vi "VFD FGV.vi"(4 "Slave ID (255)":u8, 5 "values Mutiple Reg":u16[](array[numeric]), 6 "State":T1, 7 "Coil Value":bool, 8 "error In":errorcluster, 9 "value":u16, 10 "address":u16, 11 "IP Address":string="localhost") -> (0 "error out":errorcluster, 2 "Coils":bool[](array[boolean]), 3 "Registers":u16[](array[numeric]))   [LabVIEW 2026, in "VFD Library.lvlib"]
uses:
  VFD Library.lvlib
  State Selection FGV.ctl
  <vilib>/NI/Modbus Library/API/Master/Modbus Master.lvclass
  <vilib>/NI/Modbus Library/API/Wrapper/Create TCP Master.vi
  <vilib>/NI/Modbus Library/API/Wrapper/API Main.lvlib
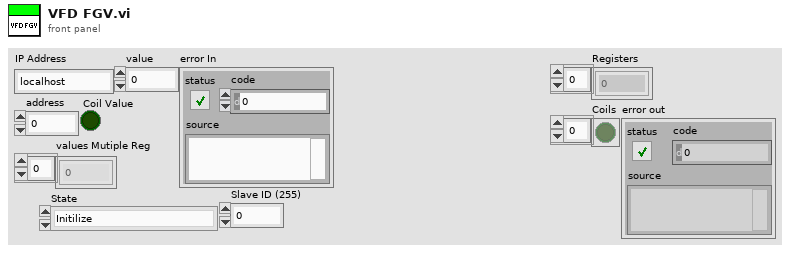
[diagram p1: front panel]
types:
  T1 = typedef "State Selection FGV.ctl" = enum16{"Initilize", "Write Reg", "Write Multiple Reg", "Read Reg", "Write Coil", "Read Coil", "Reset", "Close"}
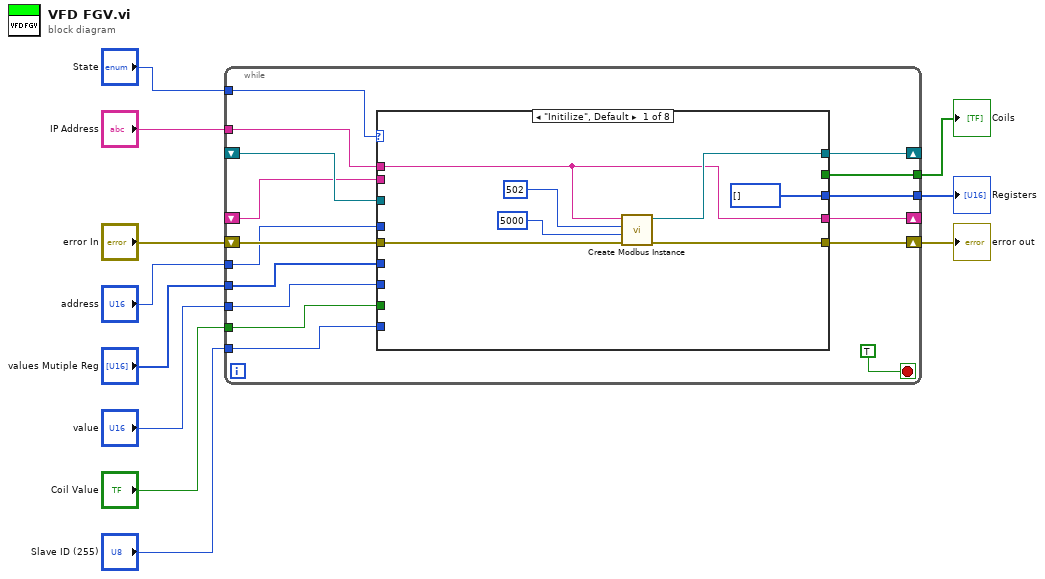
[diagram p0: block diagram]
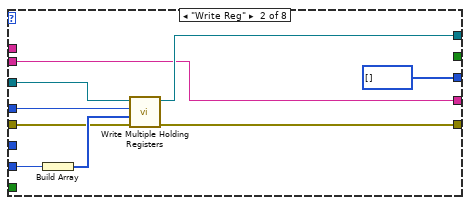
[diagram p2: hidden frame]
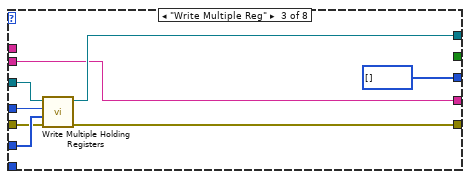
[diagram p3: hidden frame]
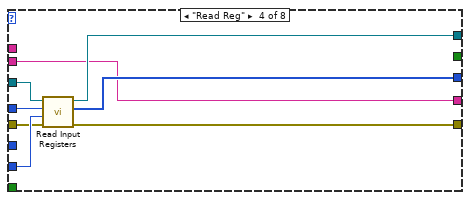
[diagram p4: hidden frame]
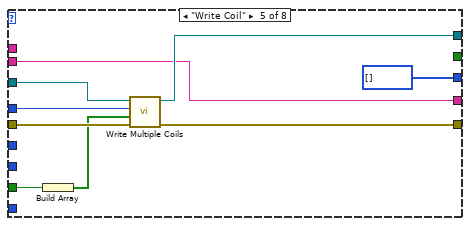
[diagram p5: hidden frame]
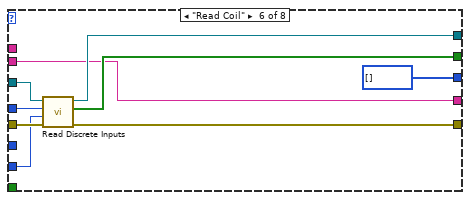
[diagram p6: hidden frame]
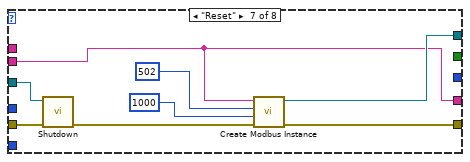
[diagram p7: hidden frame]
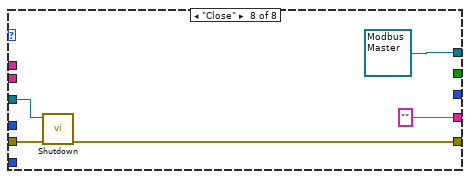
[diagram p8: hidden frame]
diagram:
  n1 = while {
    tunnel: "IP Address" -> [w26]
    shift-right: [w25] -> _
    shift-left: _ -> [w21]
    shift-right: [w24] -> w3
    shift-left: "error In" -> [w23]
    tunnel: "State" -> [w22]
    tunnel: "address" -> [w20]
    tunnel: "value" -> [w19]
    tunnel: [w18] -> w7
    tunnel: "Coil Value" -> [w17]
    tunnel: [w16] -> w5
    tunnel: "values Mutiple Reg" -> [w15]
    tunnel: "Slave ID (255)" -> [w14]
    shift-right: [w13] -> _
    shift-left: _ -> [w12]
    stop <- TRUE stop-if-true
    n2 = case shown="\"Initilize\", Default" w22 {
      tunnel: w26 -> [w28 _ _ _ _ _ _ _]
      tunnel: [w33 w38 w50 w58 w66 w75 w83 refnum<class "Modbus Master.lvclass"> refnum ("Modbus Master")] -> w25
      tunnel: [w31 w36 w45 w53 w64 w73 w82 w87] -> w24
      tunnel: w23 -> [w32 w37 w46 w55 w65 w74 w85 w88]
      tunnel: w21 -> [_ w39 w49 w59 w67 w76 w84 w89]
      tunnel: w20 -> [_ w42 w48 w57 w63 w71 _ _]
      tunnel: w19 -> [_ w41 _ w56 _ w70 _ _]
      tunnel: [u16[] [] ("Registers") u16[] [] ("Registers") u16[] [] ("Registers") w54 u16[] [] ("Registers") u16[] [] ("Registers") _ _] -> w18
      tunnel: w17 -> [_ _ _ _ w62 _ _ _]
      tunnel: [_ _ _ _ _ w72 _ _] -> w16
      tunnel: w15 -> [_ _ w47 _ _ _ _ _]
      tunnel: w14 -> [_ _ _ _ _ _ _ _]
      tunnel: [w28 w35 w44 w52 w60 w69 w79 "" ("IP Address")] -> w13
      tunnel: w12 -> [_ w35 w44 w52 w60 w69 w79 _]
      frame "Initilize", Default {
        n3 = call-poly <vilib>:"Create Modbus Instance.vi"("error in"=w32, "connect timeout ms"=5000 ("Timeout (10000)"), "port (502)"=u16 502 ("Port (502)"), "address"=w28) -> ("error out"=w31:errorcluster, "TCP master instance"=w33:refnum<class "Modbus Master.lvclass">)  [unwired: 6 in]
      }
      frame "Write Reg" {
        n4 = Build Array(w41) -> (w40:u16[])
        n5 = call-dynamic "Write Multiple Holding Registers.vi"("error in"=w37, "registers to write"=w40, "starting address"=w42, "Modbus master in"=w39) -> ("error out"=w36:errorcluster, "Modbus master out"=w38:refnum<class "Modbus Master.lvclass">)  [unwired: 6 in]
      }
      frame "Write Multiple Reg" {
        n6 = call-dynamic "Write Multiple Holding Registers.vi"("error in"=w46, "registers to write"=w47, "starting address"=w48, "Modbus master in"=w49) -> ("error out"=w45:errorcluster, "Modbus master out"=w50:refnum<class "Modbus Master.lvclass">)  [unwired: 6 in]
      }
      frame "Read Reg" {
        n7 = call-dynamic "Read Input Registers.vi"("error in"=w55, "number of inputs"=w56, "starting address"=w57, "Modbus master in"=w59) -> ("error out"=w53:errorcluster, "register values"=w54:u16[], "Modbus master out"=w58:refnum<class "Modbus Master.lvclass">)  [unwired: 5 in]
      }
      frame "Write Coil" {
        n8 = Build Array(w62) -> (w61:bool[])
        n9 = call-dynamic "Write Multiple Coils.vi"("error in"=w65, "coils to write"=w61, "starting address"=w63, "Modbus master in"=w67) -> ("error out"=w64:errorcluster, "Modbus master out"=w66:refnum<class "Modbus Master.lvclass">)  [unwired: 6 in]
      }
      frame "Read Coil" {
        n10 = call-dynamic "Read Discrete Inputs.vi"("error in"=w74, "number of inputs"=w70, "starting address"=w71, "Modbus master in"=w76) -> ("error out"=w73:errorcluster, "discrete inputs"=w72:bool[], "Modbus master out"=w75:refnum<class "Modbus Master.lvclass">)  [unwired: 5 in]
      }
      frame "Reset" {
        n11 = call-dynamic "Shutdown.vi"("error in"=w85, "Modbus master in"=w84) -> ("error out"=w81:errorcluster)  [unwired: 9 in]
        n12 = call-poly <vilib>:"Create Modbus Instance.vi"("error in"=w81, "connect timeout ms"=1000 ("Timeout (10000)"), "port (502)"=u16 502 ("Port (502)"), "address"=w79) -> ("error out"=w82:errorcluster, "TCP master instance"=w83:refnum<class "Modbus Master.lvclass">)  [unwired: 6 in]
      }
      frame "Close" {
        n13 = call-dynamic "Shutdown.vi"("error in"=w88, "Modbus master in"=w89) -> ("error out"=w87:errorcluster)  [unwired: 9 in]
      }
    }
  }
  "Registers" <- w7
  "Coils" <- w5
  "error out" <- w3
